vi "write_sub_fw3.vi"(0 "OUTSET":u16, 1 "instance":i32, 5 "OUTCLR":u16, 7 "OUTTGL":u16, 9 "AOUT Array":u16[](array[numeric]), 11 "Servo Val Array":u16[](array[numeric]), 12 "Motor Val Array":u16[](array[numeric])) -> ()   [LabVIEW 2022 SP3]
uses:
  LVLib/SADI_FW3.lvlib
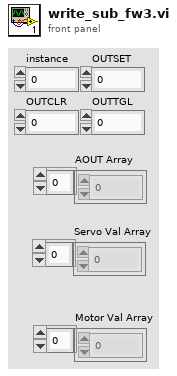
[diagram p1: front panel]
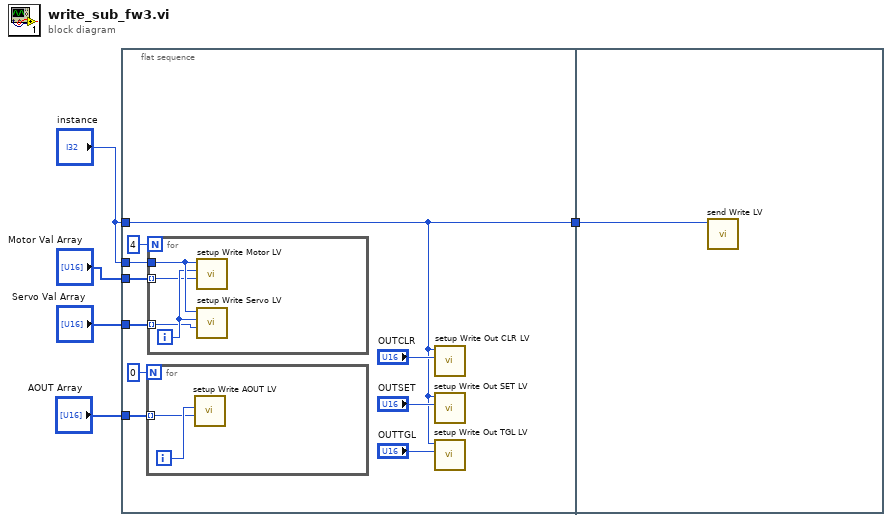
[diagram p0: block diagram]
diagram:
  n1 = flat-sequence {
    tunnel: "AOUT Array" -> [w15]
    tunnel: "instance" -> [w9]
    tunnel: "instance" -> [w6]
    tunnel: "Servo Val Array" -> [w8]
    tunnel: "Motor Val Array" -> [w7]
    tunnel: [w6] -> w1
    tunnel: w1 -> [w22]
    frame #0 {
      n2 = for {
        N: 0 -> [_]
        tunnel: w15 -> [w20] mode=indexing
        i -> [w21]
        n3 = call "setup Write AOUT LV.vi"("AOUT"=w20, "aoutNum"=w21) -> ()  [unwired: 10 in]
      }
      n4 = for {
        N: 4 -> [_]
        tunnel: w9 -> [w19]
        tunnel: w8 -> [w17] mode=indexing
        tunnel: w7 -> [w16] mode=indexing
        i -> [w18]
        n5 = call "setup Write Motor LV.vi"("value"=w16, "motorNum"=w18, "instance"=w19) -> ()  [unwired: 9 in]
        n6 = call "setup Write Servo LV.vi"("value"=w17, "servoNum"=w18, "instance"=w19) -> ()  [unwired: 9 in]
      }
      n7 = call "setup Write Out CLR LV.vi"("outMsk"="OUTCLR", "instance"=w6) -> ()  [unwired: 10 in]
      n8 = call "setup Write Out SET LV.vi"("outMsk"="OUTSET", "instance"=w6) -> ()  [unwired: 10 in]
      n9 = call "setup Write Out TGL LV.vi"("outMsk"="OUTTGL", "instance"=w6) -> ()  [unwired: 10 in]
    }
    frame #1 {
      n10 = call "send Write LV.vi"("instance"=w22) -> ()  [unwired: 11 in]
    }
  }
